vi "FunctionGenerator.vi"() -> ()   [LabVIEW 2011]
panel:
  in  "stop":bool
  in  "Offset RST":bool
  in  "Offset":dbl(knob) scale=-5.0..5.0
  out "Frequency":dbl format="%#_3pHz"
  out "Waveform 2":dynamicdata(graph) caption="DC with Uniform Noise"
  in  "Noise":dbl(knob)=0.6 caption="Noise amplitude" scale=0.0..5.0
  out "Sine":bool
  out "Square":bool
  out "Triangle":bool
  out "Sawtooth":bool
  out "DC":bool
  in  "Function":i32(knob) scale=0.0..4.0 scale format="%#_2g"
  in  "Frequency 2":dbl(knob)=10.1 caption="Frequency" scale=20.0..20000.0 scale format="%#5_2p"
  out "DC Voltage":dbl
  in  "Duty Cycle (%)":dbl(knob)=50.0 scale=0.0..100.0
  out "Amplitude":dbl format="%#_3gV"
  in  "Amplitude 2":dbl(knob)=1.0 caption="Amplitude" scale=0.0..10.0
  # "Function Generator"
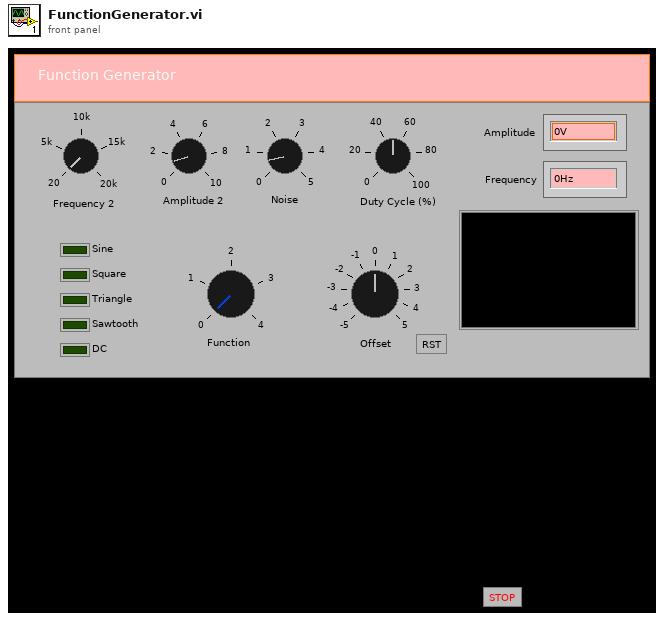
[diagram p1: front panel]
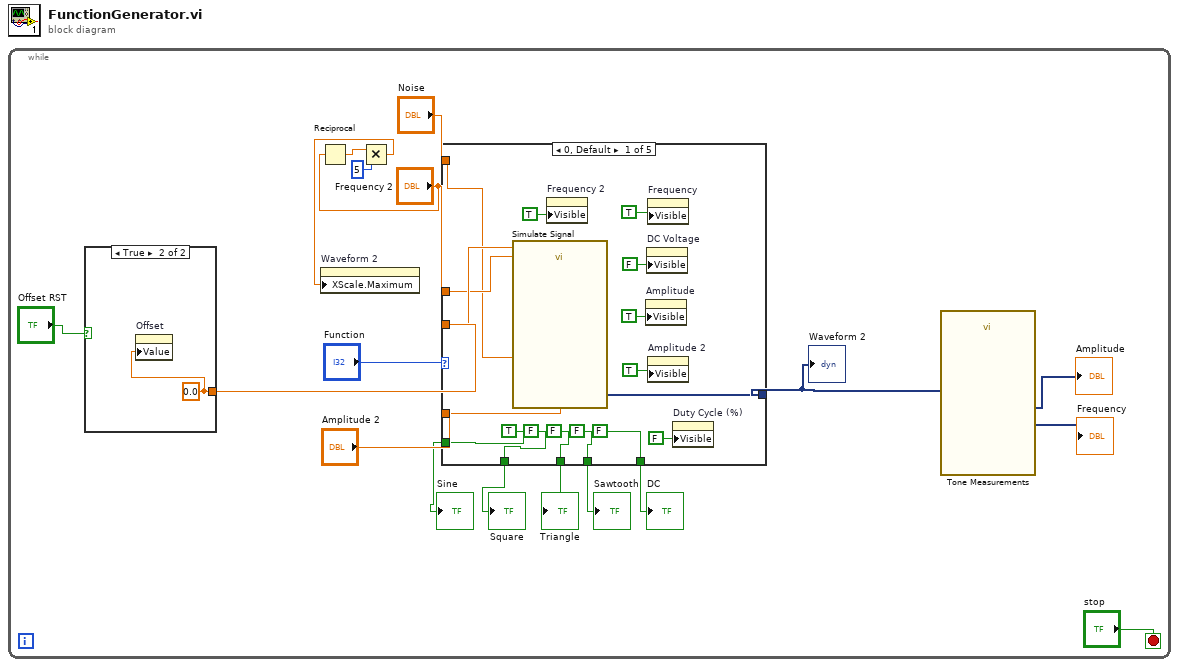
[diagram p0: block diagram]
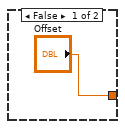
[diagram p2: hidden frame]
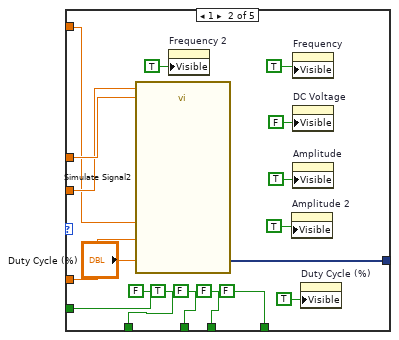
[diagram p3: hidden frame]
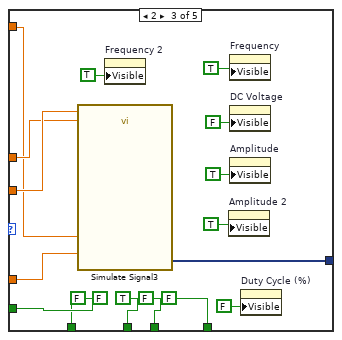
[diagram p4: hidden frame]
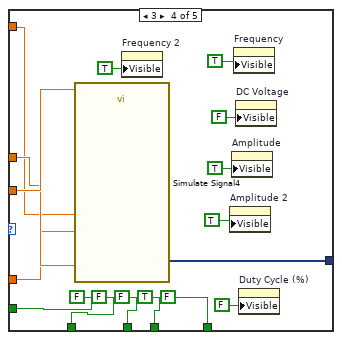
[diagram p5: hidden frame]
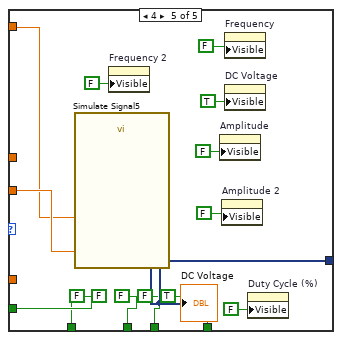
[diagram p6: hidden frame]
diagram:
  n1 = while {
    stop <- "stop" stop-if-true
    n2 = case shown="True" "Offset RST" {
      tunnel: ["Offset" w20] -> w3
      frame False {
      }
      frame True {
        w20 = 0.0 ("Offset")
        n3 = property on="Offset" class="Knob (strict)"("Value"=w20) -> ()  [unwired: 2 in, 2 out]
      }
    }
    n4 = Reciprocal(x="Frequency 2") -> (1/x=w13:dbl)
    n5 = Multiply(x=w13, y=5) -> (x*y=w12:dbl)
    n6 = property on="Waveform 2" class="WFGraph (strict)"("XScale.Maximum"=w12) -> ()  [unwired: 2 in, 2 out]
    n7 = case shown="0, Default" "Function" {
      tunnel: w3 -> [w36 w52 w69 w85 w98]
      tunnel: "Amplitude 2" -> [w35 w51 w67 w83 _]
      tunnel: [w34 w50 w66 w82 w99] -> w2
      tunnel: "Frequency 2" -> [w33 w53 w68 w84 _]
      tunnel: "Noise" -> [w32 w49 w65 w81 w97]
      tunnel: [TRUE FALSE FALSE FALSE FALSE] -> w10
      tunnel: [FALSE TRUE FALSE FALSE FALSE] -> w9
      tunnel: [FALSE FALSE TRUE FALSE FALSE] -> w8
      tunnel: [FALSE FALSE FALSE TRUE FALSE] -> w7
      tunnel: [FALSE FALSE FALSE FALSE TRUE] -> w6
      frame 0, Default {
        n8 = call "Simulate Signal"("Offset"=w36, "Frequency"=w33, "Amplitude"=w35, "Noise amplitude"=w32) -> ("Sine with Uniform Noise"=w34:dynamicdata)  [unwired: 10 in, 1 out]
        n9 = property on="Frequency 2" class="Knob (strict)"("Visible"=TRUE) -> ()  [unwired: 2 in, 2 out]
        n10 = property on="Amplitude" class="DigNum (strict)"("Visible"=TRUE) -> ()  [unwired: 2 in, 2 out]
        n11 = property on="DC Voltage" class="DigNum (strict)"("Visible"=FALSE) -> ()  [unwired: 2 in, 2 out]
        n12 = property on="Frequency" class="DigNum (strict)"("Visible"=TRUE) -> ()  [unwired: 2 in, 2 out]
        n13 = property on="Amplitude 2" class="Knob (strict)"("Visible"=TRUE) -> ()  [unwired: 2 in, 2 out]
        n14 = property on="Duty Cycle (%)" class="Knob (strict)"("Visible"=FALSE) -> ()  [unwired: 2 in, 2 out]
      }
      frame 1 {
        n15 = call "Simulate Signal2"("Offset"=w52, "Duty Cycle (%)"="Duty Cycle (%)", "Frequency"=w53, "Amplitude"=w51, "Noise amplitude"=w49) -> ("Square with Uniform Noise"=w50:dynamicdata)  [unwired: 9 in, 1 out]
        n16 = property on="Frequency 2" class="Knob (strict)"("Visible"=TRUE) -> ()  [unwired: 2 in, 2 out]
        n17 = property on="Amplitude 2" class="Knob (strict)"("Visible"=TRUE) -> ()  [unwired: 2 in, 2 out]
        n18 = property on="Frequency" class="DigNum (strict)"("Visible"=TRUE) -> ()  [unwired: 2 in, 2 out]
        n19 = property on="DC Voltage" class="DigNum (strict)"("Visible"=FALSE) -> ()  [unwired: 2 in, 2 out]
        n20 = property on="Amplitude" class="DigNum (strict)"("Visible"=TRUE) -> ()  [unwired: 2 in, 2 out]
        n21 = property on="Duty Cycle (%)" class="Knob (strict)"("Visible"=TRUE) -> ()  [unwired: 2 in, 2 out]
      }
      frame 2 {
        n22 = call "Simulate Signal3"("Offset"=w69, "Frequency"=w68, "Amplitude"=w67, "Noise amplitude"=w65) -> ("Triangle with Uniform Noise"=w66:dynamicdata)  [unwired: 10 in, 1 out]
        n23 = property on="Frequency 2" class="Knob (strict)"("Visible"=TRUE) -> ()  [unwired: 2 in, 2 out]
        n24 = property on="Amplitude 2" class="Knob (strict)"("Visible"=TRUE) -> ()  [unwired: 2 in, 2 out]
        n25 = property on="Frequency" class="DigNum (strict)"("Visible"=TRUE) -> ()  [unwired: 2 in, 2 out]
        n26 = property on="DC Voltage" class="DigNum (strict)"("Visible"=FALSE) -> ()  [unwired: 2 in, 2 out]
        n27 = property on="Amplitude" class="DigNum (strict)"("Visible"=TRUE) -> ()  [unwired: 2 in, 2 out]
        n28 = property on="Duty Cycle (%)" class="Knob (strict)"("Visible"=FALSE) -> ()  [unwired: 2 in, 2 out]
      }
      frame 3 {
        n29 = call "Simulate Signal4"("Offset"=w85, "Frequency"=w84, "Amplitude"=w83, "Noise amplitude"=w81) -> ("Sawtooth with Uniform Noise"=w82:dynamicdata)  [unwired: 10 in, 1 out]
        n30 = property on="Frequency 2" class="Knob (strict)"("Visible"=TRUE) -> ()  [unwired: 2 in, 2 out]
        n31 = property on="Amplitude 2" class="Knob (strict)"("Visible"=TRUE) -> ()  [unwired: 2 in, 2 out]
        n32 = property on="Amplitude" class="DigNum (strict)"("Visible"=TRUE) -> ()  [unwired: 2 in, 2 out]
        n33 = property on="Frequency" class="DigNum (strict)"("Visible"=TRUE) -> ()  [unwired: 2 in, 2 out]
        n34 = property on="DC Voltage" class="DigNum (strict)"("Visible"=FALSE) -> ()  [unwired: 2 in, 2 out]
        n35 = property on="Duty Cycle (%)" class="Knob (strict)"("Visible"=FALSE) -> ()  [unwired: 2 in, 2 out]
      }
      frame 4 {
        n36 = call "Simulate Signal5"("Offset"=w98, "Noise amplitude"=w97) -> ("DC with Uniform Noise"=w99:dynamicdata)  [unwired: 12 in, 1 out]
        "DC Voltage" <- w99
        n37 = property on="Frequency 2" class="Knob (strict)"("Visible"=FALSE) -> ()  [unwired: 2 in, 2 out]
        n38 = property on="Amplitude" class="DigNum (strict)"("Visible"=FALSE) -> ()  [unwired: 2 in, 2 out]
        n39 = property on="Amplitude 2" class="Knob (strict)"("Visible"=FALSE) -> ()  [unwired: 2 in, 2 out]
        n40 = property on="Frequency" class="DigNum (strict)"("Visible"=FALSE) -> ()  [unwired: 2 in, 2 out]
        n41 = property on="DC Voltage" class="DigNum (strict)"("Visible"=TRUE) -> ()  [unwired: 2 in, 2 out]
        n42 = property on="Duty Cycle (%)" class="Knob (strict)"("Visible"=FALSE) -> ()  [unwired: 2 in, 2 out]
      }
    }
    "DC" <- w6
    "Sawtooth" <- w7
    "Triangle" <- w8
    "Square" <- w9
    "Sine" <- w10
    "Waveform 2" <- w2
    n43 = call "Tone Measurements"("Signals"=w2) -> ("Frequency"=→"Frequency":dynamicdata, "Amplitude"=→"Amplitude":dynamicdata)  [unwired: 8 in, 1 out]
  }
